vi "HP Values View.vi"(11 "Model in":refnum<class "Model.lvclass">) -> ()   [LabVIEW 2016, in "M1M3SupportEUI_Views.lvlib"]
uses:
  M1M3SupportEUI_Views.lvlib
  Model/Model.lvclass
  SALLV_m1m3/DataTypes/HardpointMonitorData.ctl
  SALLV_m1m3/DataTypes/HardpointActuatorData.ctl
  SALLV_m1m3/DataTypes/logevent_HardpointActuatorInfo.ctl
  SALLV_m1m3/DataTypes/logevent_HardpointMonitorInfo.ctl
  M1M3 Support Events/M1M3 Support Events.lvclass/M1M3 Support Events.ctl
  SALLV_m1m3/DataTypes/command_EnableHardpointCorrections.ctl
  SALLV_m1m3/DataTypes/command_DisableHardpointCorrections.ctl
  SALLV_m1m3/DataTypes/command_MoveHardpointActuators.ctl
  SALLV_m1m3/DataTypes/command_StopHardpointMotion.ctl
  SALLV_m1m3/DataTypes/command_EnableHardpointChase.ctl
  SALLV_m1m3/DataTypes/command_DisableHardpointChase.ctl
  SALLV_m1m3/DataTypes/command_PositionM1M3.ctl
  SALLV_m1m3/DataTypes/command_TranslateM1M3.ctl
  M1M3 Support Events/M1M3 Support Events.lvclass
  SALLV_m1m3/SALLV_m1m3.lvlib
  <vilib>/Utility/Data Type/NI_Data Type.lvlib
panel:
  out "T6":string
  out "T5":string
  out "T4":string
  out "T3":string
  out "T2":string
  out "T1":string
  out "ForceMagnitude":dbl
  out "E6":string
  out "E5":string
  out "E4":string
  out "E3":string
  out "E2":string
  out "E1":string
  out "Monitor Info Event Time Stamp":timestamp
  in  "MonitorInfoEvent":T1={"Timestamp"=0.0, "ReferenceId[6]"=[0, 0, 0, 0, 0, 0], "ModbusSubnet[6]"=[0, 0, 0, 0, 0, 0], "ModbusAddress[6]"=[0, 0, 0, 0, 0, 0], "ILCUniqueId[6]"=[0, 0, 0, 0, 0, 0], "ILCApplicationType[6]"=[0, 0, 0, 0, 0, 0], "NetworkNodeType[6]"=[0, 0, 0, 0, 0, 0], "MajorRevision[6]"=[0, 0, 0, 0, 0, 0], "MinorRevision[6]"=[0, 0, 0, 0, 0, 0], "MezzanineUniqueId[6]"=[0, 0, 0, 0, 0, 0], "MezzanineFirmwareType[6]"=[0, 0, 0, 0, 0, 0], "MezzanineMajorRevision[6]"=[0, 0, 0, 0, 0, 0], "MezzanineMinorRevision[6]"=[0, 0, 0, 0, 0, 0], "priority"=0}
  in  "Events Data Type":string(combo)
  in  "ActuatorInfoEvent":T2
  out "Z Magnitude":sgl
  out "Y Magnitude":sgl
  out "X Magnitude":sgl
  out "Z Force":sgl
  out "Y Force":sgl
  out "X Force":sgl
  in  "StopHardpointMotion":bool
  in  "HardpointMotionButton":bool
  in  "Input 6":i32
  in  "Input 5":i32
  in  "Input 4":i32
  in  "Input 3":i32
  in  "Input 2":i32
  in  "Input 1":i32
  in  "DisableHardpointCorrectionButton":bool
  in  "DisableHardpointChaseButton":bool
  in  "TranslateHardpointsButton":bool
  in  "PositionHardpointsButton":bool
  in  "Z Rotation Input":dbl
  in  "Y Rotation Input":dbl
  in  "X Rotation Input":dbl
  in  "Z Position Input":dbl
  in  "Y Position Input":dbl
  in  "X Position Input":dbl
  in  "EnableHardpointChaseButton":bool
  in  "EnableActuatorId":string(combo)
  in  "EnableHardpointCorrectionButton":bool
  out "Actuator Info Event Time Stamp":timestamp
  out "Z Rotation":sgl
  out "Y Rotation":sgl
  out "X Rotation":sgl
  out "Z Position":sgl
  out "Y Position":sgl
  out "X Position":sgl
  in  "HardpointActuatorData":T3={"Timestamp"=0.0, "StepsQueued[6]"=[0, 0, 0, 0, 0, 0], "StepsCommanded[6]"=[0, 0, 0, 0, 0, 0], "MeasuredForce[6]"=[0.0, 0.0, 0.0, 0.0, 0.0, 0.0], "Encoder[6]"=[0, 0, 0, 0, 0, 0], "Displacement[6]"=[0.0, 0.0, 0.0, 0.0, 0.0, 0.0], "Fx"=0.0, "Fy"=0.0, "Fz"=0.0, "Mx"=0.0, "My"=0.0, "Mz"=0.0, "ForceMagnitude"=0.0, "XPosition"=0.0, "YPosition"=0.0, "ZPosition"=0.0, "XRotation"=0.0, "YRotation"=0.0, "ZRotation"=0.0}
  in  "HardpointMonitorData":T4={"Timestamp"=0.0, "BreakawayLVDT[6]"=[0.0, 0.0, 0.0, 0.0, 0.0, 0.0], "DisplacementLVDT[6]"=[0.0, 0.0, 0.0, 0.0, 0.0, 0.0], "BreakawayPressure[6]"=[0.0, 0.0, 0.0, 0.0, 0.0, 0.0], "PressureSensor1[6]"=[0.0, 0.0, 0.0, 0.0, 0.0, 0.0], "PressureSensor2[6]"=[0.0, 0.0, 0.0, 0.0, 0.0, 0.0], "PressureSensor3[6]"=[0.0, 0.0, 0.0, 0.0, 0.0, 0.0]}
  out "Actuator Data Time Stamp":timestamp
  out "Monitor Data Time Stamp":timestamp
  in  "Telemetry Data Type":string(combo)
  # "Hardpoints"
  # "Events"
  # "Commands"
  # "Position"
  # "Rotation"
  # "X"
  # "3"
  # "1"
  # "2"
  # "Y"
  # "Z"
  # "6"
  # "4"
  # "5"
  # "Current Telemetry Values"
  # "Position (m)"
  # "Rotation (rad)"
  # "Force (N)"
  # "Moments(Nm)"
  # "3"
  # "1"
  # "2"
  # "X"
  # "6"
  # "4"
  # "5"
  # "Y"
  # "Z"
  # "3"
  # "1"
  # "2"
  # "6"
  # "4"
  # "5"
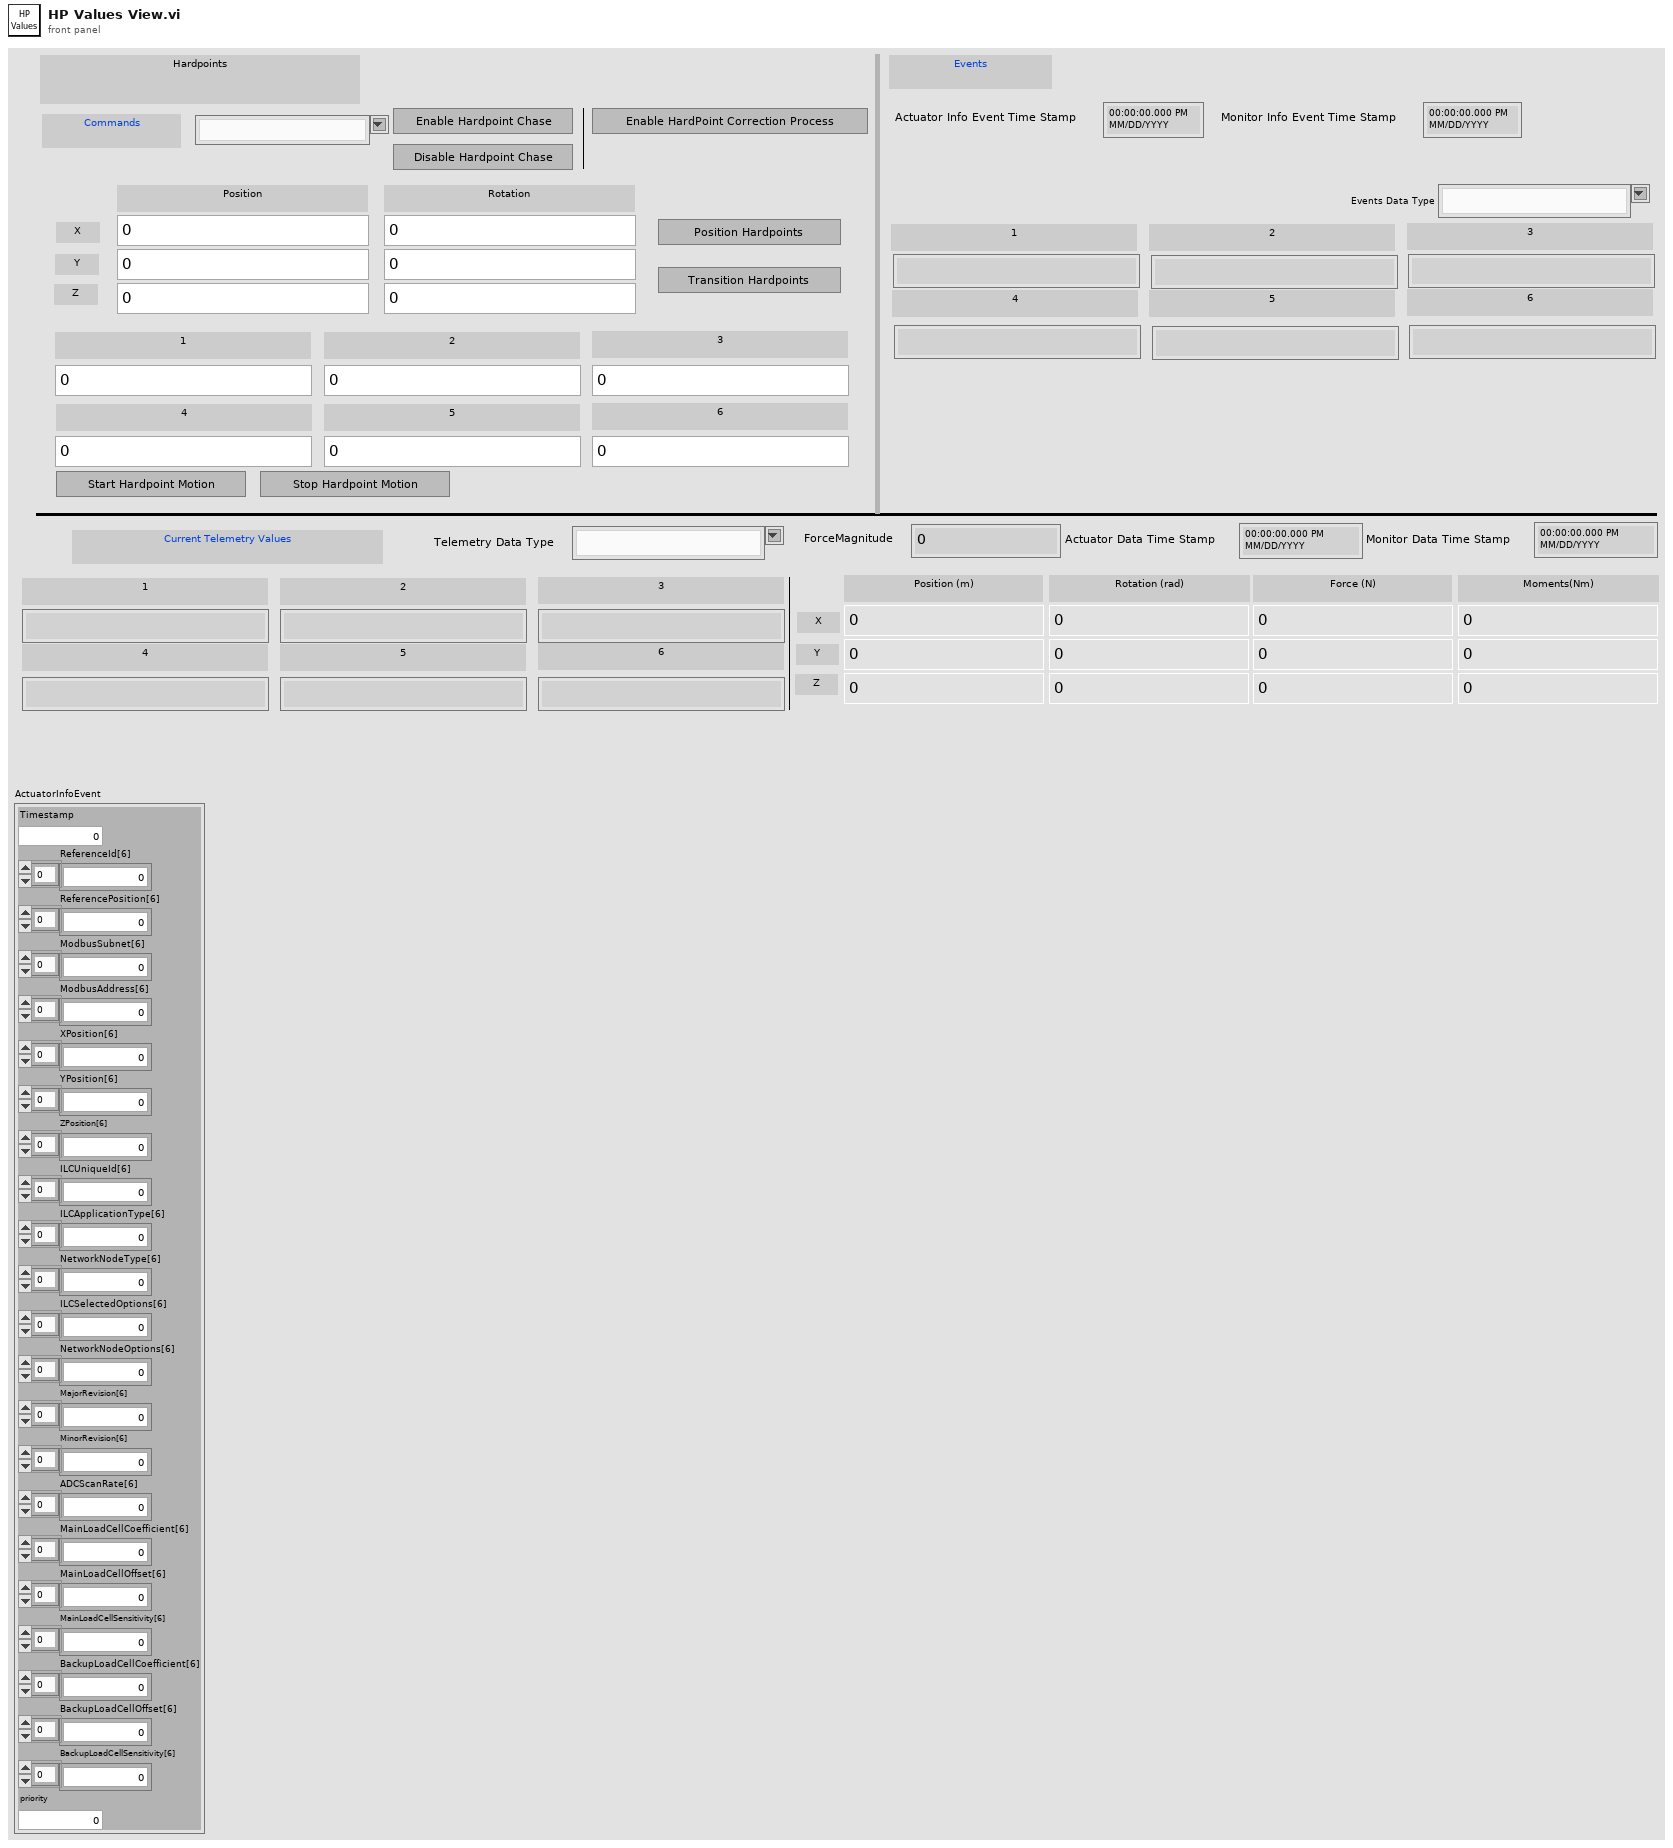
[diagram p1: front panel]
types:
  T1 = typedef "SALLV_m1m3.lvlib/logevent_HardpointMonitorInfo.ctl" = cluster{"Timestamp":dbl, "ReferenceId[6]":i16[], "ModbusSubnet[6]":i16[], "ModbusAddress[6]":i16[], "ILCUniqueId[6]":i64[], "ILCApplicationType[6]":i16[], "NetworkNodeType[6]":i16[], "MajorRevision[6]":i16[], "MinorRevision[6]":i16[], "MezzanineUniqueId[6]":i64[], "MezzanineFirmwareType[6]":i16[], "MezzanineMajorRevision[6]":i16[], "MezzanineMinorRevision[6]":i16[], "priority":i32}
  T2 = typedef "SALLV_m1m3.lvlib/logevent_HardpointActuatorInfo.ctl" = cluster{"Timestamp":dbl, "ReferenceId[6]":i16[], "ReferencePosition[6]":i32[], "ModbusSubnet[6]":i16[], "ModbusAddress[6]":i16[], "XPosition[6]":sgl[], "YPosition[6]":sgl[], "ZPosition[6]":sgl[], "ILCUniqueId[6]":i64[], "ILCApplicationType[6]":i16[], "NetworkNodeType[6]":i16[], "ILCSelectedOptions[6]":i16[], "NetworkNodeOptions[6]":i16[], "MajorRevision[6]":i16[], "MinorRevision[6]":i16[], "ADCScanRate[6]":i16[], "MainLoadCellCoefficient[6]":sgl[], "MainLoadCellOffset[6]":sgl[], "MainLoadCellSensitivity[6]":sgl[], "BackupLoadCellCoefficient[6]":sgl[], "BackupLoadCellOffset[6]":sgl[], "BackupLoadCellSensitivity[6]":sgl[], "priority":i32}
  T3 = typedef "SALLV_m1m3.lvlib/HardpointActuatorData.ctl" = cluster{"Timestamp":dbl, "StepsQueued[6]":i32[], "StepsCommanded[6]":i16[], "MeasuredForce[6]":sgl[], "Encoder[6]":i32[], "Displacement[6]":sgl[], "Fx":sgl, "Fy":sgl, "Fz":sgl, "Mx":sgl, "My":sgl, "Mz":sgl, "ForceMagnitude":sgl, "XPosition":sgl, "YPosition":sgl, "ZPosition":sgl, "XRotation":sgl, "YRotation":sgl, "ZRotation":sgl}
  T4 = typedef "SALLV_m1m3.lvlib/HardpointMonitorData.ctl" = cluster{"Timestamp":dbl, "BreakawayLVDT[6]":sgl[], "DisplacementLVDT[6]":sgl[], "BreakawayPressure[6]":sgl[], "PressureSensor1[6]":sgl[], "PressureSensor2[6]":sgl[], "PressureSensor3[6]":sgl[]}
  T5 = enum16{"", "DetailedState_DetailedStates_DisabledState", "DetailedState_DetailedStates_EnabledState", "DetailedState_DetailedStates_FaultState", "DetailedState_DetailedStates_OfflineState", "DetailedState_DetailedStates_StandbyState", "DetailedState_DetailedStates_ParkedState", "DetailedState_DetailedStates_RaisingState", "DetailedState_DetailedStates_ActiveState", "DetailedState_DetailedStates_LoweringState", "DetailedState_DetailedStates_EngineeringState", "DetailedState_DetailedStates_ParkedEngineeringState", "DetailedState_DetailedStates_RaisingEngineeringState", "DetailedState_DetailedStates_ActiveEngineeringState", "DetailedState_DetailedStates_LoweringEngineeringState", "DetailedState_DetailedStates_LoweringFaultState", "DetailedState_DetailedStates_ProfileHardpointCorrectionState"}
  T6 = typedef "M1M3SupportEUI_TypeDefs.lvlib/M1M3 Support Events.ctl" = cluster{"Inclinometer  Data":refnum<user-event>, "IMS Data":refnum<user-event>, "SAL Connected":refnum<user-event>, "Accelerometer Data":refnum<user-event>, "OuterLoop Data":refnum<user-event>, "ErrorCode Event":refnum<user-event>, "InterlockStatus Event":refnum<user-event>, "InterlockWarning Event":refnum<user-event>, "Gyro Data":refnum<user-event>, "HP Actuator Info Event":refnum<user-event>, " FA Info Event":refnum<user-event>, "HP Monitor Info Event":refnum<user-event>, "FA Data":refnum<user-event>, "HP Actuator data":refnum<user-event>, "HP Monitor data":refnum<user-event>, "Air Supply Status Event":refnum<user-event>, "Air Supply Warning Event":refnum<user-event>, "Power Data":refnum<user-event>, "PID Data":refnum<user-event>, "PID Info Event":refnum<user-event>, "Power Status Event":refnum<user-event>, "Power Supply Status Event":refnum<user-event>, "Power Warning Event":refnum<user-event>, "Summary State Event":refnum<user-event>, "Detailed State Event":refnum<user-event>, "FA Force Warning Event":refnum<user-event>, "FA Warning Event":refnum<user-event>, "FA State Event":refnum<user-event>, "Applied AberrationForces Event":refnum<user-event>, "Applied Acceleration Forcces Event":refnum<user-event>, "Applied Azimuth Forces Event":refnum<user-event>, "Applied Active Optic Forces Event":refnum<user-event>, "Applied Balance Forces Event":refnum<user-event>, "Applied Cylinder Forces Event":refnum<user-event>, "Applied Elevation Forces Event":refnum<user-event>, "Applied Forces Event":refnum<user-event>, "Applied Offset Forces Event":refnum<user-event>, "Applied Static Forces Event":refnum<user-event>, "Applied Thermal Forces Event":refnum<user-event>, "Applied Velocity Forces Event":refnum<user-event>, "Rejected Aberration Force Event":refnum<user-event>, "Rejected Acceleration Forces Event":refnum<user-event>, "Rejected Active Optic Forces Event":refnum<user-event>, "Rejected Azimuth Forces Event":refnum<user-event>, "Rejected Balance Forces Event":refnum<user-event>, "Rejected Cylinder Forces Event":refnum<user-event>, "Rejected Elevation Forces Event":refnum<user-event>, "Rejected Forces Event":refnum<user-event>, "Rejected Offset Forces Event":refnum<user-event>, "Rejected Static Forces Event":refnum<user-event>, "Rejected Thermal Forces Event":refnum<user-event>, "Rejected Velocity Forces Event":refnum<user-event>, "Command Rejection Event":refnum<user-event>, "Setting Verions Event":refnum<user-event>, "Settings Applied Event":refnum<user-event>}
  T7 = typedef "NI_Data Type.lvlib/Data Type.ctl" = enum8{"Invalid Type", "Void", "I8", "I16", "I32", "I64", "U8", "U16", "U32", "U64", "Single Float", "Double Float", "Extended Float", "Single Complex", "Double Complex", "Extended Complex", "Enum U8", "Enum U16", "Enum U32", "Enum U64", "Single Float With Unit", "Double Float With Unit", "Extended Float With Unit", "Single Complex with Unit", "Double Complex with Unit", "Extended Complex with Unit", "Boolean", "String", "Path", "Picture", "Tag", "Array", "Cluster", "Variant", "LV Variant", "Waveform", "Timestamp", "Digital Waveform", "Digital Data", "ExpressData", "Refnum", "External Data", "VI", "Poly VI", "LabVIEW Class Instance", "Fixed Point"}
  T8 = typedef "SALLV_m1m3.lvlib/command_EnableHardpointCorrections.ctl" = cluster{"EnableHardpointCorrections":bool}
  T9 = typedef "SALLV_m1m3.lvlib/command_DisableHardpointCorrections.ctl" = cluster{"DisableHardpointCorrections":bool}
  T10 = typedef "SALLV_m1m3.lvlib/command_MoveHardpointActuators.ctl" = cluster{"Steps[6]":i32[]}
  T11 = typedef "SALLV_m1m3.lvlib/command_StopHardpointMotion.ctl" = cluster{"StopHardpointMotion":bool}
  T12 = typedef "SALLV_m1m3.lvlib/command_EnableHardpointChase.ctl" = cluster{"HardpointActuator":i16}
  T13 = typedef "SALLV_m1m3.lvlib/command_DisableHardpointChase.ctl" = cluster{"HardpointActuator":i16}
  T14 = typedef "SALLV_m1m3.lvlib/command_PositionM1M3.ctl" = cluster{"XPosition":sgl, "YPosition":sgl, "ZPosition":sgl, "XRotation":sgl, "YRotation":sgl, "ZRotation":sgl}
  T15 = typedef "SALLV_m1m3.lvlib/command_TranslateM1M3.ctl" = cluster{"XTranslation":sgl, "YTranslation":sgl, "ZTranslation":sgl, "XRotation":sgl, "YRotation":sgl, "ZRotation":sgl}
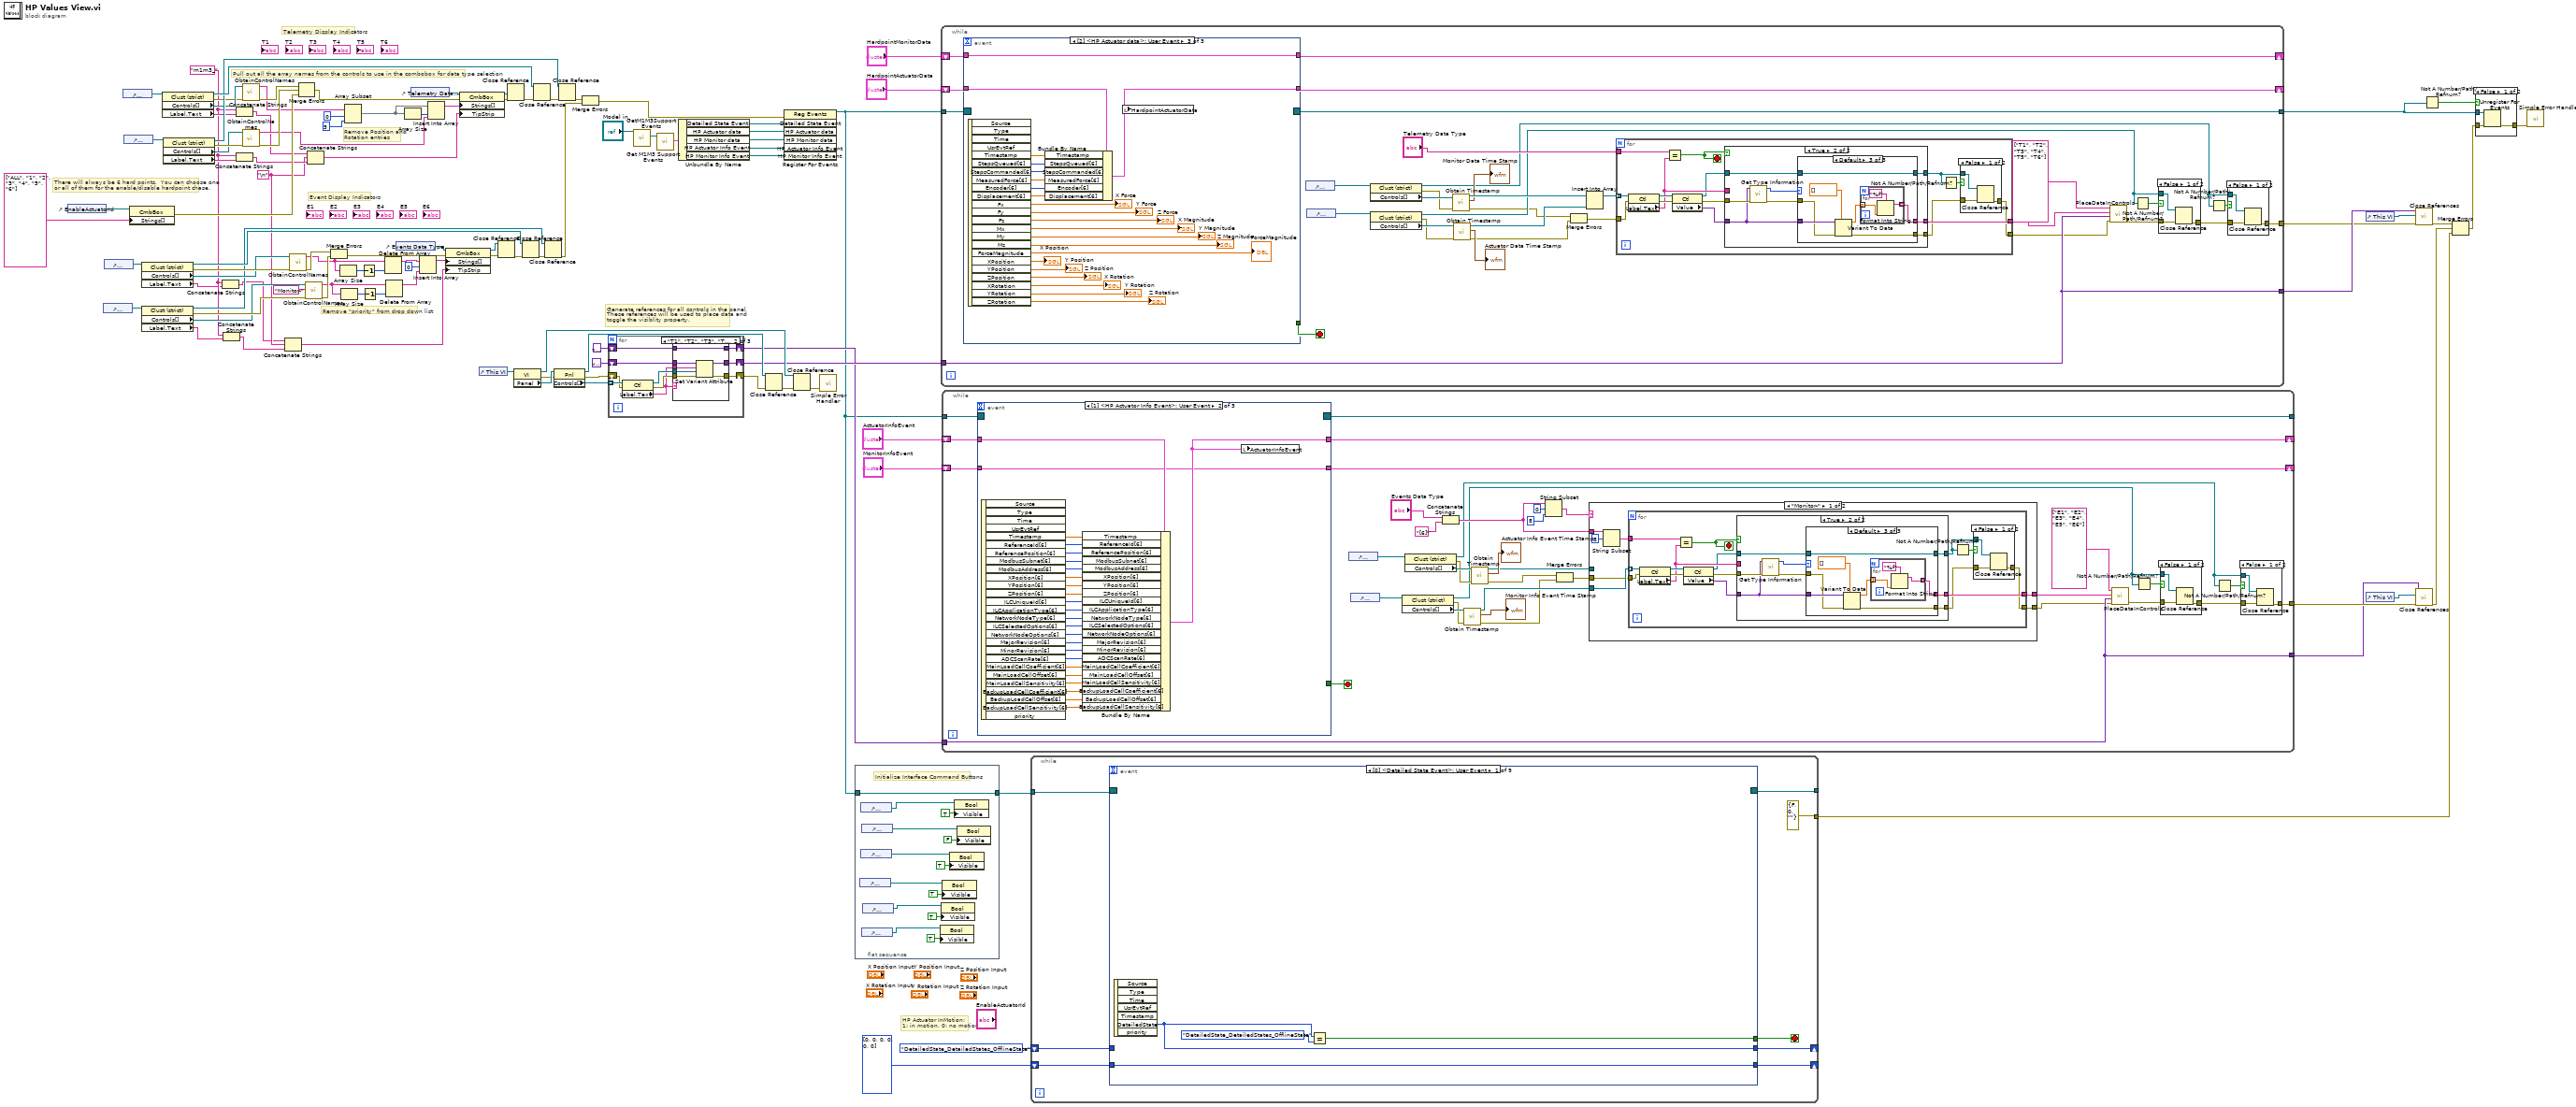
[diagram p0: block diagram]
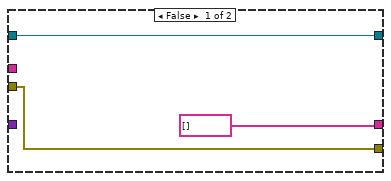
[diagram p4: hidden frame]
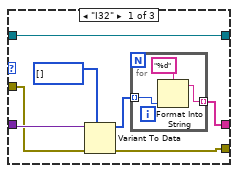
[diagram p5: hidden frame]
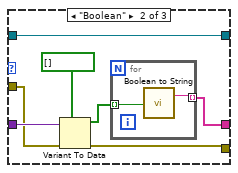
[diagram p6: hidden frame]
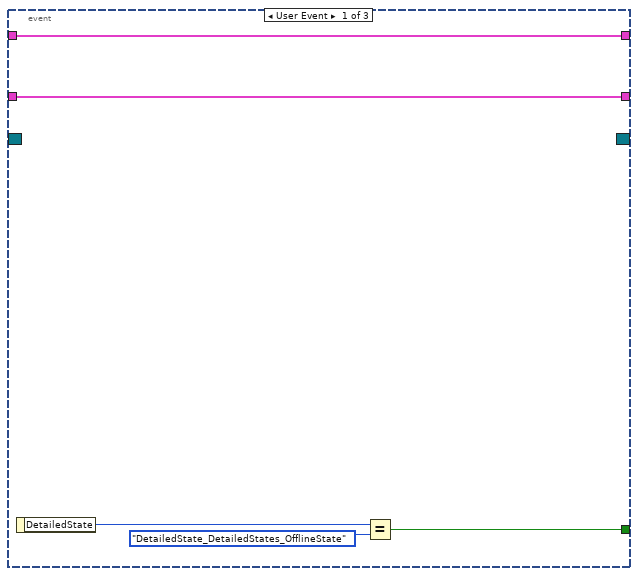
[diagram p7: hidden frame]
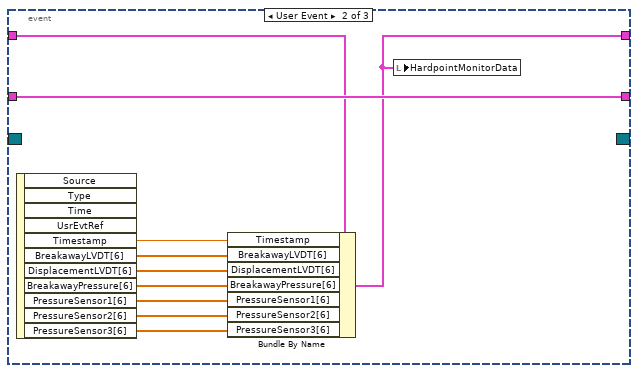
[diagram p8: hidden frame]
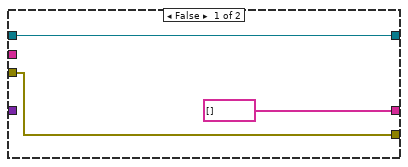
[diagram p11: hidden frame]
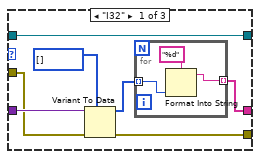
[diagram p12: hidden frame]
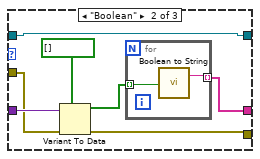
[diagram p13: hidden frame]
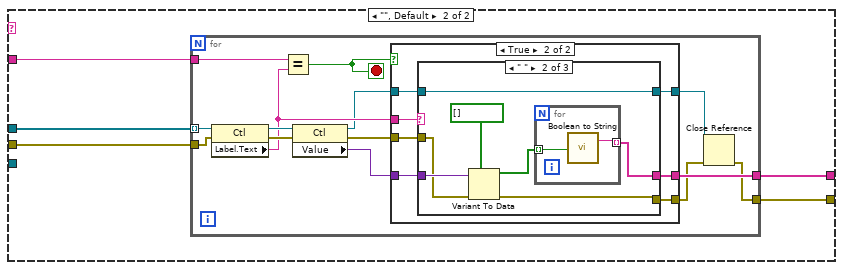
[diagram p15: hidden frame]
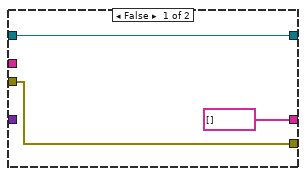
[diagram p16: hidden frame]
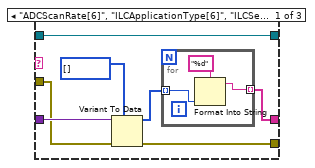
[diagram p17: hidden frame]
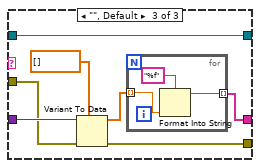
[diagram p18: hidden frame]
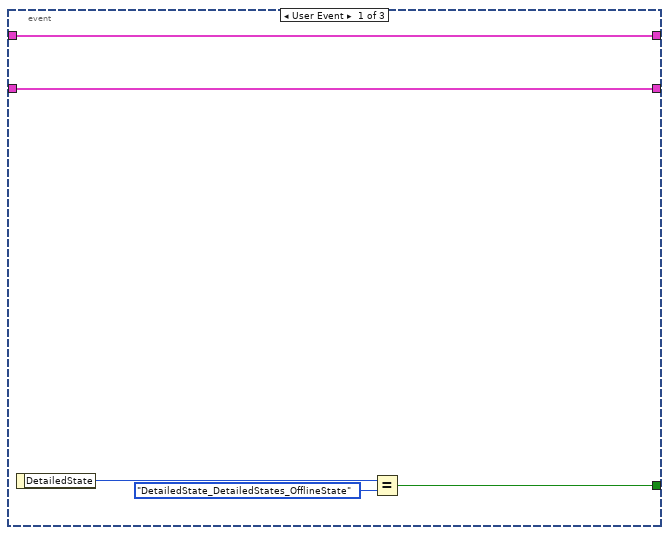
[diagram p19: hidden frame]
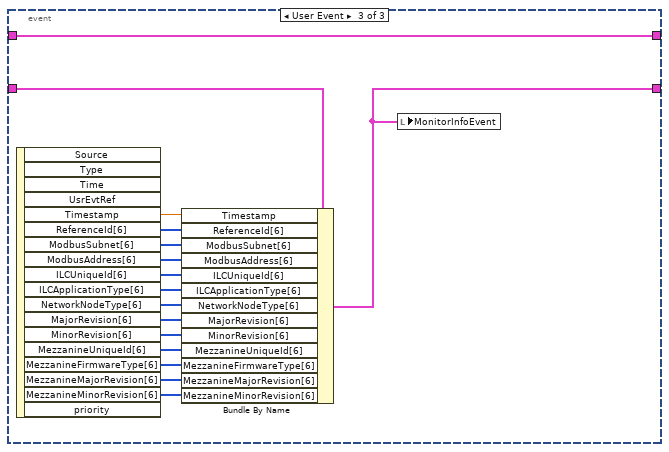
[diagram p20: hidden frame]
diagram:
  w4 = "\n"
  w8 = "m1m3_"
  # "Remove \"priority\" from drop down list"
  # "Event Display Indicators"
  # "Telemetry Display Indicators"
  # "HP Actuator InMotion:\n1: in motion, 0: no motion"
  # "There will always be 6 hard points.  You can choose one\nor all of them for the enable/disable hardpoint chase."
  # "Remove Position and\nRotation entries"
  # "Generate references for all controls in the panel\nThese references will be used to place data and\ntoggle the visiblity property."
  # "Pull out all the array names from the controls to use in the combobox for data type selection"
  n1 = control-ref of="EnableActuatorId"() -> (w83:refnum<vi>)
  n2 = control-ref of="MonitorInfoEvent"() -> (w50:refnum<vi>)
  n3 = control-ref of="ActuatorInfoEvent"() -> (w76:refnum<vi>)
  n4 = control-ref of="HardpointActuatorData"() -> (w66:refnum<vi>)
  n5 = control-ref of="HardpointMonitorData"() -> (w65:refnum<vi>)
  n6 = property class="CmbBox"(reference=w83, "Strings[]"=string[] ["ALL", "1", "2", "3", "4", "5", "6"]) -> (error out=w81:errorcluster)  [unwired: 1 in, 1 out]
  n7 = property class="Clust (strict)"(reference=w76) -> (reference out=w72:refnum<vi>, error out=w56:errorcluster, "Controls[]"=w55:refnum<vi>[], "Label.Text"=w7:string)  [unwired: 1 in]
  n8 = property class="Clust (strict)"(reference=w50) -> (reference out=w47:refnum<vi>, error out=w51:errorcluster, "Controls[]"=w49:refnum<vi>[], "Label.Text"=w6:string)  [unwired: 1 in]
  n9 = property class="Clust (strict)"(reference=w66) -> (reference out=w106:refnum<vi>, error out=w63:errorcluster, "Controls[]"=w64:refnum<vi>[], "Label.Text"=w12:string)  [unwired: 1 in]
  n10 = property class="Clust (strict)"(reference=w65) -> (reference out=w101:refnum<vi>, error out=w61:errorcluster, "Controls[]"=w60:refnum<vi>[], "Label.Text"=w11:string)  [unwired: 1 in]
  n11 = Concatenate Strings(w8, w7) -> (w3:string)
  n12 = Concatenate Strings(w8, w6) -> (w2:string)
  n13 = Concatenate Strings(w8, w12) -> (w10:string)
  n14 = Concatenate Strings(w8, w11) -> (w5:string)
  n15 = call "ObtainControlNames.vi"("error in (no error)"=w63, "ControlRefnumArray"=w64) -> ("error out"=w62:errorcluster, "ControlNamesArray"=w33:string[])  [unwired: 8 in]
  n16 = call "ObtainControlNames.vi"("error in (no error)"=w61, "ControlRefnumArray"=w60) -> ("error out"=w59:errorcluster, "ControlNamesArray"=w58:string[])  [unwired: 8 in]
  n17 = Concatenate Strings(w3, w4, w2) -> (w1:string)
  n18 = call "ObtainControlNames.vi"("error in (no error)"=w56, "ControlRefnumArray"=w55) -> ("error out"=w54:errorcluster, "ControlNamesArray"=w41:string[])  [unwired: 8 in]
  n19 = Merge Errors(w62, w59, w81) -> (w105:errorcluster)
  n20 = call "ObtainControlNames.vi"("error in (no error)"=w51, "AddedPrefix"="Monitor-", "ControlRefnumArray"=w49) -> ("error out"=w46:errorcluster, "ControlNamesArray"=w35:string[])  [unwired: 7 in]
  n21 = Concatenate Strings(w10, w4, w5) -> (w9:string)
  n22 = Merge Errors(w54, w46) -> (w73:errorcluster)
  n23 = Array Size(array=w41) -> (size(s)=w40:i32)
  n24 = Array Size(array=w35) -> (size(s)=w36:i32)
  n25 = Array Subset(array=w33, index=0, length=5 ("y")) -> (w32:string[])
  n26 = Decrement(x=w40) -> (x-1=w39:i32)
  n27 = Decrement(x=w36) -> (x-1=w37:i32)
  n28 = Delete From Array(array=w41, index=w39) -> (array with subset deleted=w38:string[])  [unwired: 1 in, 1 out]
  n29 = Delete From Array(array=w35, index=w37) -> (array with subset deleted=w34:string[])  [unwired: 1 in, 1 out]
  n30 = control-ref of="Events Data Type"() -> (w74:refnum<vi>)
  n31 = Array Size(array=w32) -> (size(s)=w85:i32)
  n32 = control-ref of="Telemetry Data Type"() -> (w100:refnum<vi>)
  n33 = Insert Into Array(array=w38, index=0, new element=w34) -> (w52:string[])
  n34 = Insert Into Array(array=w32, index=w85, new element=w58) -> (w102:string[])
  n35 = property class="CmbBox"(reference=w74, error in=w73, "Strings[]"=w52, "TipStrip"=w1) -> (reference out=w27:refnum<vi>, error out=w26:errorcluster)
  n36 = property class="CmbBox"(reference=w100, error in=w105, "Strings[]"=w102, "TipStrip"=w9) -> (reference out=w29:refnum<vi>, error out=w28:errorcluster)
  n37 = control-ref of="This VI"() -> (w87:refnum<vi>)
  n38 = Close Reference(reference=w27, error in (no error)=w26) -> (error out=w57:errorcluster)
  n39 = Close Reference(reference=w29, error in (no error)=w28) -> (error out=w103:errorcluster)
  n40 = property class="VI"(reference=w87) -> (reference out=w97:refnum<vi>, error out=w88:errorcluster, "Panel"=w89:refnum<vi>)  [unwired: 1 in]
  n41 = Close Reference(reference=w72, error in (no error)=w57) -> (error out=w48:errorcluster)
  n42 = Close Reference(reference=w106, error in (no error)=w103) -> (error out=w104:errorcluster)
  n43 = Close Reference(reference=w47, error in (no error)=w48) -> (error out=w43:errorcluster)
  n44 = property class="Pnl"(reference=w89, error in=w88) -> (reference out=w95:refnum<vi>, error out=w92:errorcluster, "Controls[]"=w90:refnum<vi>[])
  n45 = Close Reference(reference=w101, error in (no error)=w104) -> (error out=w45:errorcluster)
  n46 = Merge Errors(w45, w43) -> (w44:errorcluster)
  n47 = for {
    tunnel: w90 -> [w121] mode=indexing
    shift-right: [w118] -> w77
    shift-left: variant -> [w120]
    shift-right: [w115] -> w94
    shift-left: w92 -> [w117]
    shift-right: [w113] -> w71
    shift-left: variant -> [w114]
    n48 = property class="Ctl"(reference=w121, error in=w117) -> (reference out=w119:refnum<vi>, error out=w116:errorcluster, "Label.Text"=w112:string)
    n49 = case shown="\"T1\", \"T2\", \"T3\", \"T4\", \"T5\", \"T6\"" w112 {
      tunnel: w120 -> [w123 w131 w136]
      tunnel: w112 -> [_ w130 w135]
      tunnel: w119 -> [_ w129 w134]
      tunnel: [w123 w128 w136] -> w118
      tunnel: w116 -> [w122 w127 w133]
      tunnel: [w122 w126 w132] -> w115
      tunnel: w114 -> [w124 w125 w138]
      tunnel: [w124 w125 w137] -> w113
      frame "", Default {
      }
      frame "T1", "T2", "T3", "T4", "T5", "T6" {
        n50 = Set Variant Attribute(Variant=w131, name=w130, value=w129, error in=w127) -> (Variant out=w128:variant, error out=w126:errorcluster)  [unwired: 1 out]
      }
      frame "E1", "E2", "E3", "E4", "E5", "E6" {
        n51 = Set Variant Attribute(Variant=w138, name=w135, value=w134, error in=w133) -> (Variant out=w137:variant, error out=w132:errorcluster)  [unwired: 1 out]
      }
    }
  }
  n52 = call "GetM1M3SupportEvents.vi"("Model in"="Model in") -> ("M1M3 Support Events out"=w111:refnum<class "M1M3 Support Events.lvclass">)  [unwired: 8 in, 2 out]
  n53 = call "Get M1M3 Support Events.vi"("M1M3 Support Events in"=w111) -> ("M1M3 Support Events"=w110:T6)  [unwired: 9 in, 1 out]
  n54 = Unbundle By Name(w110) -> ("Detailed State Event"=w108:refnum<user-event>, "HP Actuator data"=w107:refnum<user-event>, "HP Monitor data"=w86:refnum<user-event>, "HP Actuator Info Event"=w84:refnum<user-event>, "HP Monitor Info Event"=w80:refnum<user-event>)
  n55 = Close Reference(reference=w95, error in (no error)=w94) -> (error out=w93:errorcluster)
  n56 = register-events(error in=w44, w108, w107, w86, w84, w80) -> (reference out=w70:refnum<event-registration>)  [unwired: 1 in, 1 out]
  n57 = Close Reference(reference=w97, error in (no error)=w93) -> (error out=w96:errorcluster)
  n58 = call <vilib>:"Simple Error Handler.vi"("error in (no error)"=w96) -> ()  [unwired: 4 in, 5 out]
  n59 = flat-sequence {
    tunnel: [w151] -> w78
    tunnel: w70 -> [w151]
    frame #0 {
      # "Initialize Interface Command Buttons"
      n60 = control-ref of="DisableHardpointChaseButton"() -> (w139:refnum<vi>)
      n61 = control-ref of="EnableHardpointCorrectionButton"() -> (w144:refnum<vi>)
      n62 = control-ref of="EnableHardpointChaseButton"() -> (w141:refnum<vi>)
      n63 = control-ref of="StopHardpointMotion"() -> (w148:refnum<vi>)
      n64 = control-ref of="DisableHardpointCorrectionButton"() -> (w143:refnum<vi>)
      n65 = control-ref of="HardpointMotionButton"() -> (w147:refnum<vi>)
      n66 = property class="Bool"(reference=w148, "Visible"=TRUE) -> ()  [unwired: 1 in, 2 out]
      n67 = property class="Bool"(reference=w147, "Visible"=TRUE) -> ()  [unwired: 1 in, 2 out]
      n68 = property class="Bool"(reference=w139, "Visible"=TRUE) -> ()  [unwired: 1 in, 2 out]
      n69 = property class="Bool"(reference=w141, "Visible"=TRUE) -> ()  [unwired: 1 in, 2 out]
      n70 = property class="Bool"(reference=w144, "Visible"=TRUE) -> ()  [unwired: 1 in, 2 out]
      n71 = property class="Bool"(reference=w143, "Visible"=FALSE) -> ()  [unwired: 1 in, 2 out]
    }
  }
  n72 = while {
    tunnel: w70 -> [w184]
    shift-right: [w181] -> _
    shift-left: "HardpointMonitorData" -> [w182]
    shift-right: [w179] -> _
    shift-left: "HardpointActuatorData" -> [w180]
    tunnel: w77 -> [w162]
    tunnel: [w162] -> w25
    tunnel: [w176] -> w17
    tunnel: [w156] -> w19
    stop <- w183 stop-if-true
    n73 = event shown="[2] <HP Actuator data>: User Event" {
      selector: w184 -> [_ _ _]
      dyn-events: [_ _ _] -> w176
      timeout: _ -> [_ _ _]
      tunnel: [w248 _ _] -> w183
      tunnel: w182 -> [w247 w257 w280]
      tunnel: [w247 w256 w280] -> w181
      tunnel: w180 -> [w246 w258 w279]
      tunnel: [w246 w258 w278] -> w179
      event User Event {
        n74 = event-data() -> ("DetailedState"=w245:T5)  [unwired: 1 in]
        n75 = Equal?(x=w245, y=T5."DetailedState_DetailedStates_OfflineState") -> (x = y?=w248:bool)
      }
      event User Event {
        n76 = event-data() -> ("Timestamp"=w255:dbl, "BreakawayLVDT[6]"=w254:sgl[], "DisplacementLVDT[6]"=w253:sgl[], "BreakawayPressure[6]"=w252:sgl[], "PressureSensor1[6]"=w251:sgl[], "PressureSensor2[6]"=w250:sgl[], "PressureSensor3[6]"=w249:sgl[])  [unwired: 1 in, 4 out]
        n77 = Bundle By Name(cluster=w257, "Timestamp"=w255, "BreakawayLVDT[6]"=w254, "DisplacementLVDT[6]"=w253, "BreakawayPressure[6]"=w252, "PressureSensor1[6]"=w251, "PressureSensor2[6]"=w250, "PressureSensor3[6]"=w249) -> (w256:T4)
        n78 = local write "HardpointMonitorData"(w256) -> ()
      }
      event User Event {
        n79 = event-data() -> ("Timestamp"=w277:dbl, "StepsQueued[6]"=w276:i32[], "StepsCommanded[6]"=w275:i16[], "MeasuredForce[6]"=w274:sgl[], "Encoder[6]"=w273:i32[], "Displacement[6]"=w272:sgl[], "Fx"=→"X Force":sgl, "Fy"=→"Y Force":sgl, "Fz"=→"Z Force":sgl, "Mx"=→"X Magnitude":sgl, "My"=→"Y Magnitude":sgl, "Mz"=→"Z Magnitude":sgl, "ForceMagnitude"=→"ForceMagnitude":sgl, "XPosition"=→"X Position":sgl, "YPosition"=→"Y Position":sgl, "ZPosition"=→"Z Position":sgl, "XRotation"=→"X Rotation":sgl, "YRotation"=→"Y Rotation":sgl, "ZRotation"=→"Z Rotation":sgl)  [unwired: 1 in, 4 out]
        n80 = Bundle By Name(cluster=w279, "Timestamp"=w277, "StepsQueued[6]"=w276, "StepsCommanded[6]"=w275, "MeasuredForce[6]"=w274, "Encoder[6]"=w273, "Displacement[6]"=w272) -> (w278:T3)
        n81 = local write "HardpointActuatorData"(w278) -> ()
      }
    }
    n82 = control-ref of="HardpointMonitorData"() -> (w178:refnum<vi>)
    n83 = control-ref of="HardpointActuatorData"() -> (w177:refnum<vi>)
    n84 = property class="Clust (strict)"(reference=w178) -> (reference out=w157:refnum<vi>, error out=w171:errorcluster, "Controls[]"=w173:refnum<vi>[])  [unwired: 1 in]
    n85 = property class="Clust (strict)"(reference=w177) -> (reference out=w160:refnum<vi>, error out=w169:errorcluster, "Controls[]"=w170:refnum<vi>[])  [unwired: 1 in]
    n86 = call "Obtain Timestamp.vi"("error in (no error)"=w171, "ControlRefnumArray"=w173) -> ("error out"=w154:errorcluster, "Time Stamp"=→"Monitor Data Time Stamp":timestamp, "Array"=w172:refnum<vi>[])  [unwired: 7 in]
    n87 = call "Obtain Timestamp.vi"("error in (no error)"=w169, "ControlRefnumArray"=w170) -> ("error out"=w153:errorcluster, "Time Stamp"=→"Actuator Data Time Stamp":timestamp, "Array"=w166:refnum<vi>[])  [unwired: 7 in]
    n88 = Merge Errors(w154, w153) -> (w152:errorcluster)
    n89 = Insert Into Array(array=w172, new element=w166) -> (w174:refnum<vi>[])  [unwired: 1 in]
    n90 = for {
      tunnel: "Telemetry Data Type" -> [w193]
      tunnel: w174 -> [w198] mode=indexing
      tunnel: [w191] -> w164
      tunnel: [w186] -> w155
      tunnel: w152 -> [w185]
      stop <- w195 stop-if-true
      n91 = property class="Ctl"(reference=w198, error in=w185) -> (reference out=w196:refnum<vi>, error out=w197:errorcluster, "Label.Text"=w192:string)
      n92 = Equal?(x=w193, y=w192) -> (x = y?=w195:bool)
      n93 = property class="Ctl"(reference=w196, error in=w197) -> (reference out=w190:refnum<vi>, error out=w194:errorcluster, "Value"=w199:variant)
      n94 = case shown="True" w195 {
        tunnel: w199 -> [_ w208]
        tunnel: w192 -> [_ _]
        tunnel: w194 -> [w206 w210]
        tunnel: [w206 w214] -> w187
        tunnel: [string[] [] w213] -> w191
        tunnel: w190 -> [w204 w212]
        tunnel: [w204 w211] -> w188
        frame False {
        }
        frame True {
          n95 = call <vilib>:"Get Type Information.vi"("error in (no error)"=w210, "Variant"=w208) -> ("error out"=w209:errorcluster, "Type"=w207:T7)  [unwired: 5 in, 3 out]
          n96 = case shown="Default" w207 {
            tunnel: w208 -> [w220 w230 w240]
            tunnel: [w216 w226 w235] -> w213
            tunnel: w209 -> [w219 w229 w238]
            tunnel: [w218 w228 w237] -> w214
            tunnel: w212 -> [w215 w225 w234]
            tunnel: [w215 w225 w234] -> w211
            frame "I32" {
              n97 = Variant To Data(error in=w219, type=i32[] [], Variant=w220) -> (data=w217:i32[], error out=w218:errorcluster)
              n98 = for {
                tunnel: w217 -> [w224] mode=indexing
                tunnel: [w223] -> w216 mode=indexing
                n99 = Format Into String(format string="%d", w224) -> (resulting string=w223:string)  [unwired: 2 in, 1 out]
              }
            }
            frame "Boolean" {
              n100 = Variant To Data(error in=w229, type=bool[] [], Variant=w230) -> (data=w227:bool[], error out=w228:errorcluster)
              n101 = for {
                tunnel: w227 -> [w233] mode=indexing
                tunnel: [w232] -> w226 mode=indexing
                n102 = call "Boolean to String.vi"("BooleanValue"=w233) -> ("StringForm"=w232:string)  [unwired: 1 out]
              }
            }
            frame Default {
              n103 = Variant To Data(error in=w238, type=dbl[] [], Variant=w240) -> (data=w236:dbl[], error out=w237:errorcluster)
              n104 = for {
                tunnel: w236 -> [w243] mode=indexing
                tunnel: [w242] -> w235 mode=indexing
                n105 = Format Into String(format string="%f", w243) -> (resulting string=w242:string)  [unwired: 2 in, 1 out]
              }
            }
          }
        }
      }
      n106 = Not A Number/Path/Refnum?(number/path/refnum=w188) -> (NaN/Path/Refnum?=w189:bool)
      n107 = case shown="False" w189 {
        tunnel: w187 -> [w202 w203]
        tunnel: [w201 w203] -> w186
        tunnel: w188 -> [w200 _]
        frame False {
          n108 = Close Reference(reference=w200, error in (no error)=w202) -> (error out=w201:errorcluster)
        }
        frame True {
        }
      }
    }
    n109 = call "PlaceDataInControls.vi"("error in (no error)"=w155, "Variant"=w162, "DataArray"=w164, "ControlNamesArray"=string[] ["T1", "T2", "T3", "T4", "T5", "T6"]) -> ("error out"=w161:errorcluster)  [unwired: 7 in]
    n110 = Not A Number/Path/Refnum?(number/path/refnum=w160) -> (NaN/Path/Refnum?=w163:bool)
    n111 = case shown="False" w163 {
      tunnel: w161 -> [w283 w284]
      tunnel: [w282 w284] -> w158
      tunnel: w160 -> [w281 _]
      frame False {
        n112 = Close Reference(reference=w281, error in (no error)=w283) -> (error out=w282:errorcluster)
      }
      frame True {
      }
    }
    n113 = Not A Number/Path/Refnum?(number/path/refnum=w157) -> (NaN/Path/Refnum?=w159:bool)
    n114 = case shown="False" w159 {
      tunnel: w158 -> [w287 w288]
      tunnel: [w286 w288] -> w156
      tunnel: w157 -> [w285 _]
      frame False {
        n115 = Close Reference(reference=w285, error in (no error)=w287) -> (error out=w286:errorcluster)
      }
      frame True {
      }
    }
  }
  n116 = while {
    tunnel: w71 -> [w307]
    tunnel: w70 -> [w325]
    shift-right: [w322] -> _
    shift-left: "ActuatorInfoEvent" -> [w323]
    shift-right: [w317] -> _
    shift-left: "MonitorInfoEvent" -> [w318]
    tunnel: [w295] -> w22
    tunnel: [w307] -> w21
    tunnel: [w289] -> _
    stop <- w324 stop-if-true
    n117 = event shown="[1] <HP Actuator Info Event>: User Event" {
      selector: w325 -> [_ _ _]
      dyn-events: [_ _ _] -> w289
      timeout: _ -> [_ _ _]
      tunnel: [w454 _ _] -> w324
      tunnel: w323 -> [w453 w479 w495]
      tunnel: [w453 w478 w495] -> w322
      tunnel: w318 -> [w452 w455 w494]
      tunnel: [w452 w455 w493] -> w317
      event User Event {
        n118 = event-data() -> ("DetailedState"=w451:T5)  [unwired: 1 in]
        n119 = Equal?(x=w451, y=T5."DetailedState_DetailedStates_OfflineState") -> (x = y?=w454:bool)
      }
      event User Event {
        n120 = event-data() -> ("Timestamp"=w477:dbl, "ReferenceId[6]"=w476:i16[], "ReferencePosition[6]"=w475:i32[], "ModbusSubnet[6]"=w474:i16[], "ModbusAddress[6]"=w473:i16[], "XPosition[6]"=w472:sgl[], "YPosition[6]"=w471:sgl[], "ZPosition[6]"=w470:sgl[], "ILCUniqueId[6]"=w469:i64[], "ILCApplicationType[6]"=w468:i16[], "NetworkNodeType[6]"=w467:i16[], "ILCSelectedOptions[6]"=w466:i16[], "NetworkNodeOptions[6]"=w465:i16[], "MajorRevision[6]"=w464:i16[], "MinorRevision[6]"=w463:i16[], "ADCScanRate[6]"=w462:i16[], "MainLoadCellCoefficient[6]"=w461:sgl[], "MainLoadCellOffset[6]"=w460:sgl[], "MainLoadCellSensitivity[6]"=w459:sgl[], "BackupLoadCellCoefficient[6]"=w458:sgl[], "BackupLoadCellOffset[6]"=w457:sgl[], "BackupLoadCellSensitivity[6]"=w456:sgl[])  [unwired: 1 in, 5 out]
        n121 = Bundle By Name(cluster=w479, "Timestamp"=w477, "ReferenceId[6]"=w476, "ReferencePosition[6]"=w475, "ModbusSubnet[6]"=w474, "ModbusAddress[6]"=w473, "XPosition[6]"=w472, "YPosition[6]"=w471, "ZPosition[6]"=w470, "ILCUniqueId[6]"=w469, "ILCApplicationType[6]"=w468, "NetworkNodeType[6]"=w467, "ILCSelectedOptions[6]"=w466, "NetworkNodeOptions[6]"=w465, "MajorRevision[6]"=w464, "MinorRevision[6]"=w463, "ADCScanRate[6]"=w462, "MainLoadCellCoefficient[6]"=w461, "MainLoadCellOffset[6]"=w460, "MainLoadCellSensitivity[6]"=w459, "BackupLoadCellCoefficient[6]"=w458, "BackupLoadCellOffset[6]"=w457, "BackupLoadCellSensitivity[6]"=w456) -> (w478:T2)
        n122 = local write "ActuatorInfoEvent"(w478) -> ()
      }
      event User Event {
        n123 = event-data() -> ("Timestamp"=w492:dbl, "ReferenceId[6]"=w491:i16[], "ModbusSubnet[6]"=w490:i16[], "ModbusAddress[6]"=w489:i16[], "ILCUniqueId[6]"=w488:i64[], "ILCApplicationType[6]"=w487:i16[], "NetworkNodeType[6]"=w486:i16[], "MajorRevision[6]"=w485:i16[], "MinorRevision[6]"=w484:i16[], "MezzanineUniqueId[6]"=w483:i64[], "MezzanineFirmwareType[6]"=w482:i16[], "MezzanineMajorRevision[6]"=w481:i16[], "MezzanineMinorRevision[6]"=w480:i16[])  [unwired: 1 in, 5 out]
        n124 = Bundle By Name(cluster=w494, "Timestamp"=w492, "ReferenceId[6]"=w491, "ModbusSubnet[6]"=w490, "ModbusAddress[6]"=w489, "ILCUniqueId[6]"=w488, "ILCApplicationType[6]"=w487, "NetworkNodeType[6]"=w486, "MajorRevision[6]"=w485, "MinorRevision[6]"=w484, "MezzanineUniqueId[6]"=w483, "MezzanineFirmwareType[6]"=w482, "MezzanineMajorRevision[6]"=w481, "MezzanineMinorRevision[6]"=w480) -> (w493:T1)
        n125 = local write "MonitorInfoEvent"(w493) -> ()
      }
    }
    n126 = control-ref of="ActuatorInfoEvent"() -> (w321:refnum<vi>)
    n127 = control-ref of="MonitorInfoEvent"() -> (w312:refnum<vi>)
    n128 = property class="Clust (strict)"(reference=w312) -> (reference out=w296:refnum<vi>, error out=w309:errorcluster, "Controls[]"=w313:refnum<vi>[])  [unwired: 1 in]
    n129 = property class="Clust (strict)"(reference=w321) -> (reference out=w294:refnum<vi>, error out=w315:errorcluster, "Controls[]"=w316:refnum<vi>[])  [unwired: 1 in]
    n130 = Concatenate Strings("Events Data Type", "[6]" ("string")) -> (w305:string)
    n131 = call "Obtain Timestamp.vi"("error in (no error)"=w309, "ControlRefnumArray"=w313) -> ("error out"=w292:errorcluster, "Time Stamp"=→"Monitor Info Event Time Stamp":timestamp, "Array"=w301:refnum<vi>[])  [unwired: 7 in]
    n132 = call "Obtain Timestamp.vi"("error in (no error)"=w315, "ControlRefnumArray"=w316) -> ("error out"=w293:errorcluster, "Time Stamp"=→"Actuator Info Event Time Stamp":timestamp, "Array"=w310:refnum<vi>[])  [unwired: 7 in]
    n133 = String Subset(string=w305, offset (0)=0, length (rest)=8 ("length (rest)")) -> (substring=w304:string)
    n134 = Merge Errors(w293, w292) -> (w291:errorcluster)
    n135 = case shown="\"Monitor-\"" w304 {
      tunnel: w310 -> [_ w396]
      tunnel: [w328 w395] -> w306
      tunnel: w305 -> [w332 w394]
      tunnel: w301 -> [w329 _]
      tunnel: w291 -> [w326 w393]
      tunnel: [w327 w392] -> w290
      frame "Monitor-" {
        n136 = String Subset(string=w332, offset (0)=8) -> (substring=w330:string)  [unwired: 1 in]
        n137 = for {
          tunnel: w330 -> [w341]
          tunnel: w329 -> [w346] mode=indexing
          tunnel: [w334] -> w327
          tunnel: [w339] -> w328
          tunnel: w326 -> [w337]
          stop <- w343 stop-if-true
          n138 = property class="Ctl"(reference=w346, error in=w337) -> (reference out=w344:refnum<vi>, error out=w345:errorcluster, "Label.Text"=w340:string)
          n139 = Equal?(x=w341, y=w340) -> (x = y?=w343:bool)
          n140 = property class="Ctl"(reference=w344, error in=w345) -> (reference out=w338:refnum<vi>, error out=w342:errorcluster, "Value"=w347:variant)
          n141 = case shown="True" w343 {
            tunnel: w347 -> [_ w352]
            tunnel: w340 -> [_ _]
            tunnel: w342 -> [w350 w354]
            tunnel: [w350 w358] -> w335
            tunnel: [string[] [] w357] -> w339
            tunnel: w338 -> [w348 w356]
            tunnel: [w348 w355] -> w333
            frame False {
            }
            frame True {
              n142 = call <vilib>:"Get Type Information.vi"("error in (no error)"=w354, "Variant"=w352) -> ("error out"=w353:errorcluster, "Type"=w351:T7)  [unwired: 5 in, 3 out]
              n143 = case shown="Default" w351 {
                tunnel: w352 -> [w364 w374 w384]
                tunnel: [w360 w370 w379] -> w357
                tunnel: w353 -> [w363 w373 w382]
                tunnel: [w362 w372 w381] -> w358
                tunnel: w356 -> [w359 w369 w378]
                tunnel: [w359 w369 w378] -> w355
                frame "I32" {
                  n144 = Variant To Data(error in=w363, type=i32[] [], Variant=w364) -> (data=w361:i32[], error out=w362:errorcluster)
                  n145 = for {
                    tunnel: w361 -> [w366] mode=indexing
                    tunnel: [w367] -> w360 mode=indexing
                    n146 = Format Into String(format string="%d", w366) -> (resulting string=w367:string)  [unwired: 2 in, 1 out]
                  }
                }
                frame "Boolean" {
                  n147 = Variant To Data(error in=w373, type=bool[] [], Variant=w374) -> (data=w371:bool[], error out=w372:errorcluster)
                  n148 = for {
                    tunnel: w371 -> [w377] mode=indexing
                    tunnel: [w376] -> w370 mode=indexing
                    n149 = call "Boolean to String.vi"("BooleanValue"=w377) -> ("StringForm"=w376:string)  [unwired: 1 out]
                  }
                }
                frame Default {
                  n150 = Variant To Data(error in=w382, type=dbl[] [], Variant=w384) -> (data=w380:dbl[], error out=w381:errorcluster)
                  n151 = for {
                    tunnel: w380 -> [w386] mode=indexing
                    tunnel: [w385] -> w379 mode=indexing
                    n152 = Format Into String(format string="%f", w386) -> (resulting string=w385:string)  [unwired: 2 in, 1 out]
                  }
                }
              }
            }
          }
          n153 = Not A Number/Path/Refnum?(number/path/refnum=w333) -> (NaN/Path/Refnum?=w336:bool)
          n154 = case shown="False" w336 {
            tunnel: w335 -> [w390 w391]
            tunnel: [w389 w391] -> w334
            tunnel: w333 -> [w388 _]
            frame False {
              n155 = Close Reference(reference=w388, error in (no error)=w390) -> (error out=w389:errorcluster)
            }
            frame True {
            }
          }
        }
      }
      frame "", Default {
        n156 = for {
          tunnel: w394 -> [w404]
          tunnel: w396 -> [w409] mode=indexing
          tunnel: [w398] -> w392
          tunnel: [w402] -> w395
          tunnel: w393 -> [w397]
          stop <- w406 stop-if-true
          n157 = property class="Ctl"(reference=w409, error in=w397) -> (reference out=w407:refnum<vi>, error out=w408:errorcluster, "Label.Text"=w403:string)
          n158 = Equal?(x=w404, y=w403) -> (x = y?=w406:bool)
          n159 = property class="Ctl"(reference=w407, error in=w408) -> (reference out=w401:refnum<vi>, error out=w405:errorcluster, "Value"=w410:variant)
          n160 = case shown="True" w406 {
            tunnel: w410 -> [_ w420]
            tunnel: w403 -> [_ w419]
            tunnel: w405 -> [w413 w418]
            tunnel: [w413 w417] -> w399
            tunnel: [string[] [] w416] -> w402
            tunnel: w401 -> [w411 w415]
            tunnel: [w411 w414] -> w400
            frame False {
            }
            frame True {
              n161 = case shown="\" \"" w419 {
                tunnel: w420 -> [w426 w436 w446]
                tunnel: [w422 w432 w441] -> w416
                tunnel: w418 -> [w425 w435 w444]
                tunnel: [w424 w434 w443] -> w417
                tunnel: w415 -> [w421 w431 w440]
                tunnel: [w421 w431 w440] -> w414
                frame "ADCScanRate[6]", "ILCApplicationType[6]", "ILCSelectedOptions[6]", "ILCUniqueId[6]", "MajorRevision[6]", "MinorRevision[6]", "ModbusAddress[6]", "ModbusSubnet[6]" {
                  n162 = Variant To Data(error in=w425, type=i32[] [], Variant=w426) -> (data=w423:i32[], error out=w424:errorcluster)
                  n163 = for {
                    tunnel: w423 -> [w429] mode=indexing
                    tunnel: [w428] -> w422 mode=indexing
                    n164 = Format Into String(format string="%d", w429) -> (resulting string=w428:string)  [unwired: 2 in, 1 out]
                  }
                }
                frame " " {
                  n165 = Variant To Data(error in=w435, type=bool[] [], Variant=w436) -> (data=w433:bool[], error out=w434:errorcluster)
                  n166 = for {
                    tunnel: w433 -> [w439] mode=indexing
                    tunnel: [w438] -> w432 mode=indexing
                    n167 = call "Boolean to String.vi"("BooleanValue"=w439) -> ("StringForm"=w438:string)  [unwired: 1 out]
                  }
                }
                frame "", Default {
                  n168 = Variant To Data(error in=w444, type=dbl[] [], Variant=w446) -> (data=w442:dbl[], error out=w443:errorcluster)
                  n169 = for {
                    tunnel: w442 -> [w449] mode=indexing
                    tunnel: [w448] -> w441 mode=indexing
                    n170 = Format Into String(format string="%f", w449) -> (resulting string=w448:string)  [unwired: 2 in, 1 out]
                  }
                }
              }
            }
          }
          n171 = Close Reference(reference=w400, error in (no error)=w399) -> (error out=w398:errorcluster)
        }
      }
    }
    n172 = call "PlaceDataInControls.vi"("error in (no error)"=w290, "Variant"=w307, "DataArray"=w306, "ControlNamesArray"=string[] ["E1", "E2", "E3", "E4", "E5", "E6"]) -> ("error out"=w297:errorcluster)  [unwired: 7 in]
    n173 = Not A Number/Path/Refnum?(number/path/refnum=w296) -> (NaN/Path/Refnum?=w298:bool)
    n174 = case shown="False" w298 {
      tunnel: w297 -> [w502 w503]
      tunnel: [w501 w503] -> w300
      tunnel: w296 -> [w500 _]
      frame False {
        n175 = Close Reference(reference=w500, error in (no error)=w502) -> (error out=w501:errorcluster)
      }
      frame True {
      }
    }
    n176 = Not A Number/Path/Refnum?(number/path/refnum=w294) -> (NaN/Path/Refnum?=w299:bool)
    n177 = case shown="False" w299 {
      tunnel: w300 -> [w498 w499]
      tunnel: [w497 w499] -> w295
      tunnel: w294 -> [w496 _]
      frame False {
        n178 = Close Reference(reference=w496, error in (no error)=w498) -> (error out=w497:errorcluster)
      }
      frame True {
      }
    }
  }
  n179 = while {
    tunnel: w78 -> [w511]
    tunnel: [w509] -> _
    shift-right: [w507] -> _
    shift-left: i32[] [0, 0, 0, 0, 0, 0] -> [w508]
    shift-right: [w505] -> _
    shift-left: T5."DetailedState_DetailedStates_OfflineState" ("y") -> [w506]
    tunnel: [errorcluster {"status"=FALSE, "code"=0, "source"=""} ("error constant")] -> w13
    stop <- w510 stop-if-true
    n180 = event shown="[0] <Detailed State Event>: User Event" {
      selector: w511 -> [_ _ _ _ _ _ _ _ _]
      dyn-events: [_ _ _ _ _ _ _ _ _] -> w509
      timeout: _ -> [_ _ _ _ _ _ _ _ _]
      tunnel: [w515 _ _ _ _ _ _ _ _] -> w510
      tunnel: w508 -> [w514 w519 w535 w552 w582 w590 w616 w648 w674]
      tunnel: [w514 w519 w535 w552 w582 w590 w616 w648 w674] -> w507
      tunnel: w506 -> [_ w520 w536 w554 w581 w592 w618 w653 w679]
      tunnel: [w512 w520 w536 w554 w581 w592 w618 w653 w679] -> w505
      event User Event {
        n181 = event-data() -> ("DetailedState"=w512:T5)  [unwired: 1 in, 6 out]
        n182 = Equal?(x=w512, y=T5."DetailedState_DetailedStates_OfflineState") -> (x = y?=w515:bool)
      }
      event "EnableHardpointCorrectionButton": Value Change {
        n183 = event-data() -> ()  [unwired: 1 in, 1 out]
        n184 = control-ref of="EnableHardpointCorrectionButton"() -> (w521:refnum<vi>)
        n185 = control-ref of="DisableHardpointCorrectionButton"() -> (w517:refnum<vi>)
        n186 = Equal?(x=T5."DetailedState_DetailedStates_ActiveEngineeringState", y=w520) -> (x = y?=w523:bool)
        n187 = And(x="EnableHardpointCorrectionButton", y=w523) -> (x .and. y?=w518:bool)
        n188 = case shown="True" w518 {
          tunnel: w521 -> [_ w532]
          tunnel: w517 -> [_ w531]
          frame False {
            # "State error that action is unavailable as system is not in \nActive Engineering State"
          }
          frame True {
            n189 = call "m1m3_issueCommand_EnableHardpointCorrections.vi"("command_EnableHardpointCorrections_Ctl"=T8 {"EnableHardpointCorrections"=TRUE}) -> ("error out"=w528:errorcluster, "function return"=w525:i32)  [unwired: 8 in, 1 out]
            n190 = property class="Bool"(reference=w532, "Visible"=FALSE) -> ()  [unwired: 1 in, 2 out]
            n191 = property class="Bool"(reference=w531, "Visible"=TRUE) -> ()  [unwired: 1 in, 2 out]
            n192 = Bundle By Name(cluster=cluster{"cmdSeqNum":i32, "timeout":u32} {"cmdSeqNum"=0, "timeout"=100} ("waitComplete_Ctl"), "cmdSeqNum"=w525) -> (w524:cluster{"cmdSeqNum":i32, "timeout":u32})
            n193 = call "m1m3_waitForCompletion_EnableHardpointCorrections.vi"("error in (no error)"=w528, "waitComplete_Ctl"=w524) -> ("error out"=w527:errorcluster)  [unwired: 7 in, 2 out]
            n194 = call <vilib>:"Simple Error Handler.vi"("error in (no error)"=w527) -> ()  [unwired: 4 in, 5 out]
          }
        }
      }
      event "DisableHardpointCorrectionButton": Value Change {
        n195 = event-data() -> ()  [unwired: 1 in, 1 out]
        n196 = control-ref of="EnableHardpointCorrectionButton"() -> (w537:refnum<vi>)
        n197 = control-ref of="DisableHardpointCorrectionButton"() -> (w538:refnum<vi>)
        n198 = Equal?(x=T5."DetailedState_DetailedStates_ActiveEngineeringState", y=w536) -> (x = y?=w541:bool)
        n199 = And(x="DisableHardpointCorrectionButton", y=w541) -> (x .and. y?=w539:bool)
        n200 = case shown="True" w539 {
          tunnel: w538 -> [_ w547]
          tunnel: w537 -> [_ w545]
          frame False {
          }
          frame True {
            n201 = call "m1m3_issueCommand_DisableHardpointCorrections.vi"("command_DisableHardpointCorrections_Ctl"=T9 {"DisableHardpointCorrections"=TRUE}) -> ("error out"=w550:errorcluster, "function return"=w543:i32)  [unwired: 8 in, 1 out]
            n202 = property class="Bool"(reference=w545, "Visible"=TRUE) -> ()  [unwired: 1 in, 2 out]
            n203 = property class="Bool"(reference=w547, "Visible"=FALSE) -> ()  [unwired: 1 in, 2 out]
            n204 = Bundle By Name(cluster=cluster{"cmdSeqNum":i32, "timeout":u32} {"cmdSeqNum"=0, "timeout"=100} ("waitComplete_Ctl"), "cmdSeqNum"=w543) -> (w542:cluster{"cmdSeqNum":i32, "timeout":u32})
            n205 = call "m1m3_waitForCompletion_DisableHardpointCorrections.vi"("error in (no error)"=w550, "waitComplete_Ctl"=w542) -> ("error out"=w549:errorcluster)  [unwired: 7 in, 2 out]
            n206 = call <vilib>:"Simple Error Handler.vi"("error in (no error)"=w549) -> ()  [unwired: 4 in, 5 out]
          }
        }
      }
      event "HardpointMotionButton": Value Change {
        n207 = event-data() -> ()  [unwired: 1 in, 1 out]
        n208 = case shown="True" "HardpointMotionButton" {
          frame False {
          }
          frame True {
            # "command_MoveHardpointActuators_Ctl"
            n209 = Insert Into Array(array=i32[] [], index=0, new element="Input 1") -> (w574:i32[])
            n210 = Insert Into Array(array=w574, index=1, new element="Input 2") -> (w572:i32[])
            n211 = Insert Into Array(array=w572, index=2, new element="Input 3") -> (w570:i32[])
            n212 = Insert Into Array(array=w570, index=3, new element="Input 4") -> (w568:i32[])
            n213 = Insert Into Array(array=w568, index=4, new element="Input 5") -> (w566:i32[])
            n214 = Insert Into Array(array=w566, index=5, new element="Input 6") -> (w560:i32[])
            n215 = Bundle By Name(cluster=T10 {"Steps[6]"=[0, 0, 0, 0, 0, 0]} ("command_MoveHardpointActuators_Ctl"), "Steps[6]"=w560) -> (w579:T10)
            n216 = call "m1m3_issueCommand_MoveHardpointActuators.vi"("command_MoveHardpointActuators_Ctl"=w579) -> ("error out"=w558:errorcluster, "function return"=w556:i32)  [unwired: 8 in, 1 out]
            n217 = Bundle By Name(cluster=cluster{"cmdSeqNum":i32, "timeout":u32} {"cmdSeqNum"=0, "timeout"=100} ("waitComplete_Ctl"), "cmdSeqNum"=w556) -> (w555:cluster{"cmdSeqNum":i32, "timeout":u32})
            n218 = call "m1m3_waitForCompletion_MoveHardpointActuators.vi"("error in (no error)"=w558, "waitComplete_Ctl"=w555) -> ("error out"=w559:errorcluster)  [unwired: 7 in, 2 out]
            n219 = call <vilib>:"Simple Error Handler.vi"("error in (no error)"=w559) -> ()  [unwired: 4 in, 5 out]
          }
        }
      }
      event "StopHardpointMotion": Value Change {
        n220 = event-data() -> ()  [unwired: 1 in, 6 out]
        n221 = case shown="True" "StopHardpointMotion" {
          frame False {
          }
          frame True {
            n222 = call "m1m3_issueCommand_StopHardpointMotion.vi"("command_StopHardpointMotion_Ctl"=T11 {"StopHardpointMotion"=TRUE}) -> ("error out"=w584:errorcluster, "function return"=w586:i32)  [unwired: 8 in, 1 out]
            n223 = Bundle By Name(cluster=cluster{"cmdSeqNum":i32, "timeout":u32} {"cmdSeqNum"=0, "timeout"=100} ("waitComplete_Ctl"), "cmdSeqNum"=w586) -> (w585:cluster{"cmdSeqNum":i32, "timeout":u32})
            n224 = call "m1m3_waitForCompletion_StopHardpointMotion.vi"("error in (no error)"=w584, "waitComplete_Ctl"=w585) -> ("error out"=w588:errorcluster)  [unwired: 7 in, 2 out]
            n225 = call <vilib>:"Simple Error Handler.vi"("error in (no error)"=w588) -> ()  [unwired: 4 in, 5 out]
          }
        }
      }
      event "EnableHardpointChaseButton": Value Change {
        n226 = event-data() -> ()  [unwired: 1 in, 6 out]
        n227 = local read "EnableActuatorId"() -> (w591:string)
        n228 = case shown="True" "EnableHardpointChaseButton" {
          tunnel: w591 -> [_ w594]
          frame False {
          }
          frame True {
            n229 = case shown="\"1\", Default" w594 {
              selector: w594 -> [w606 _]
              tunnel: i32[] [] -> [w608 w610]
              tunnel: [w607 w609] -> w595
              frame "1", Default {
                n230 = Decimal String To Number(string=w606) -> (number=w605:i32)  [unwired: 2 in, 1 out]
                n231 = Insert Into Array(array=w608, new element=w605) -> (w607:i32[])  [unwired: 1 in]
              }
              frame "ALL" {
                n232 = for {
                  N: 6 -> [_]
                  shift-right: [w614] -> w609
                  shift-left: w610 -> [w615]
                  i -> [w612]
                  n233 = Increment(x=w612) -> (x+1=w613:i32)
                  n234 = Insert Into Array(array=w615, index=w612, new element=w613) -> (w614:i32[])
                }
              }
            }
            n235 = for {
              tunnel: w595 -> [w604] mode=indexing
              n236 = Bundle By Name(cluster=T12 {"HardpointActuator"=0} ("command_EnableHardpointChase_Ctl"), "HardpointActuator"=w604) -> (w602:T12)
              n237 = call "m1m3_issueCommand_EnableHardpointChase.vi"("command_EnableHardpointChase_Ctl"=w602) -> ("error out"=w597:errorcluster, "function return"=w599:i32)  [unwired: 8 in, 1 out]
              n238 = Bundle By Name(cluster=cluster{"cmdSeqNum":i32, "timeout":u32} {"cmdSeqNum"=0, "timeout"=100} ("waitComplete_Ctl"), "cmdSeqNum"=w599) -> (w598:cluster{"cmdSeqNum":i32, "timeout":u32})
              n239 = call "m1m3_waitForCompletion_EnableHardpointChase.vi"("error in (no error)"=w597, "waitComplete_Ctl"=w598) -> ("error out"=w601:errorcluster)  [unwired: 7 in, 2 out]
              n240 = call <vilib>:"Simple Error Handler.vi"("error in (no error)"=w601) -> ()  [unwired: 4 in, 5 out]
            }
          }
        }
      }
      event "DisableHardpointChaseButton": Value Change {
        n241 = event-data() -> ()  [unwired: 1 in, 6 out]
        n242 = local read "EnableActuatorId"() -> (w617:string)
        n243 = case shown="True" "DisableHardpointChaseButton" {
          tunnel: w617 -> [_ w620]
          frame False {
          }
          frame True {
            n244 = case shown="\"1\", Default" w620 {
              selector: w620 -> [w624 _]
              tunnel: i32[] [] -> [w626 w628]
              tunnel: [w625 w627] -> w621
              frame "1", Default {
                n245 = Decimal String To Number(string=w624) -> (number=w623:i32)  [unwired: 2 in, 1 out]
                n246 = Insert Into Array(array=w626, new element=w623) -> (w625:i32[])  [unwired: 1 in]
              }
              frame "ALL" {
                n247 = for {
                  N: 6 -> [_]
                  shift-right: [w632] -> w627
                  shift-left: w628 -> [w633]
                  i -> [w630]
                  n248 = Increment(x=w630) -> (x+1=w631:i32)
                  n249 = Insert Into Array(array=w633, index=w630, new element=w631) -> (w632:i32[])
                }
              }
            }
            n250 = for {
              tunnel: w621 -> [w639] mode=indexing
              n251 = Bundle By Name(cluster=T13 {"HardpointActuator"=0} ("command_DisableHardpointChase_Ctl"), "HardpointActuator"=w639) -> (w640:T13)
              n252 = call "m1m3_issueCommand_DisableHardpointChase.vi"("command_DisableHardpointChase_Ctl"=w640) -> ("error out"=w634:errorcluster, "function return"=w636:i32)  [unwired: 8 in, 1 out]
              n253 = Bundle By Name(cluster=cluster{"cmdSeqNum":i32, "timeout":u32} {"cmdSeqNum"=0, "timeout"=100} ("waitComplete_Ctl"), "cmdSeqNum"=w636) -> (w635:cluster{"cmdSeqNum":i32, "timeout":u32})
              n254 = call "m1m3_waitForCompletion_DisableHardpointChase.vi"("error in (no error)"=w634, "waitComplete_Ctl"=w635) -> ("error out"=w638:errorcluster)  [unwired: 7 in, 2 out]
              n255 = call <vilib>:"Simple Error Handler.vi"("error in (no error)"=w638) -> ()  [unwired: 4 in, 5 out]
            }
          }
        }
      }
      event "PositionHardpointsButton": Value Change {
        n256 = event-data() -> ()  [unwired: 1 in, 1 out]
        n257 = for {
          tunnel: w648 -> [w658] mode=indexing
          shift-right: [w654] -> w650
          shift-left: TRUE -> [w655]
          n258 = Equal?(x=0, y=w658) -> (x = y?=w656:bool)
          n259 = And(x=w655, y=w656) -> (x .and. y?=w654:bool)
        }
        n260 = local read "X Position Input"() -> (w647:dbl)
        n261 = local read "Y Position Input"() -> (w646:dbl)
        n262 = local read "Z Position Input"() -> (w645:dbl)
        n263 = local read "X Rotation Input"() -> (w644:dbl)
        n264 = local read "Y Rotation Input"() -> (w643:dbl)
        n265 = local read "Z Rotation Input"() -> (w642:dbl)
        n266 = And(x="PositionHardpointsButton", y=w650) -> (x .and. y?=w651:bool)
        n267 = case shown="True" w651 {
          tunnel: w644 -> [_ w664]
          tunnel: w643 -> [_ w662]
          tunnel: w642 -> [_ w663]
          tunnel: w647 -> [_ w666]
          tunnel: w646 -> [_ w659]
          tunnel: w645 -> [_ w665]
          frame False {
            # "Send error message that not all \nHP are still"
          }
          frame True {
            n268 = Bundle By Name(cluster=T14 {"XPosition"=0.0, "YPosition"=0.0, "ZPosition"=0.0, "XRotation"=0.0, "YRotation"=0.0, "ZRotation"=0.0} ("command_PositionM1M3_Ctl"), "XPosition"=w666, "YPosition"=w659, "ZPosition"=w665, "XRotation"=w664, "YRotation"=w662, "ZRotation"=w663) -> (w660:T14)
            n269 = call "m1m3_issueCommand_PositionM1M3.vi"("command_PositionM1M3_Ctl"=w660) -> ("error out"=w661:errorcluster)  [unwired: 8 in, 2 out]
            n270 = call <vilib>:"Simple Error Handler.vi"("error in (no error)"=w661) -> ()  [unwired: 4 in, 5 out]
          }
        }
      }
      event "TranslateHardpointsButton": Value Change {
        n271 = event-data() -> ()  [unwired: 1 in, 1 out]
        n272 = for {
          tunnel: w674 -> [w684] mode=indexing
          shift-right: [w680] -> w677
          shift-left: TRUE -> [w681]
          n273 = Equal?(x=0, y=w684) -> (x = y?=w682:bool)
          n274 = And(x=w681, y=w682) -> (x .and. y?=w680:bool)
        }
        n275 = local read "Y Position Input"() -> (w672:dbl)
        n276 = local read "X Rotation Input"() -> (w670:dbl)
        n277 = local read "Y Rotation Input"() -> (w669:dbl)
        n278 = local read "X Position Input"() -> (w673:dbl)
        n279 = local read "Z Position Input"() -> (w671:dbl)
        n280 = local read "Z Rotation Input"() -> (w668:dbl)
        n281 = And(x="TranslateHardpointsButton", y=w677) -> (x .and. y?=w675:bool)
        n282 = case shown="True" w675 {
          tunnel: w673 -> [_ w691]
          tunnel: w672 -> [_ w690]
          tunnel: w671 -> [_ w689]
          tunnel: w670 -> [_ w688]
          tunnel: w668 -> [_ w687]
          tunnel: w669 -> [_ w686]
          frame False {
            # "Send error message that not all HP\nare still, so not possible"
          }
          frame True {
            n283 = Bundle By Name(cluster=T15 {"XTranslation"=0.0, "YTranslation"=0.0, "ZTranslation"=0.0, "XRotation"=0.0, "YRotation"=0.0, "ZRotation"=0.0} ("command_TranslateM1M3_Ctl"), "XTranslation"=w691, "YTranslation"=w690, "ZTranslation"=w689, "XRotation"=w688, "YRotation"=w686, "ZRotation"=w687) -> (w685:T15)
            n284 = call "m1m3_issueCommand_TranslateM1M3.vi"("command_TranslateM1M3_Ctl"=w685) -> ("error out"=w693:errorcluster)  [unwired: 8 in, 2 out]
            n285 = call <vilib>:"Simple Error Handler.vi"("error in (no error)"=w693) -> ()  [unwired: 4 in, 5 out]
          }
        }
      }
    }
  }
  n286 = control-ref of="This VI"() -> (w24:refnum<vi>)
  n287 = control-ref of="This VI"() -> (w23:refnum<vi>)
  n288 = call "Close References.vi"("error in (no error)"=w19, "VI Refnum"=w24, "Variant"=w25) -> ("error out"=w67:errorcluster)  [unwired: 8 in]
  n289 = call "Close References.vi"("error in (no error)"=w22, "VI Refnum"=w23, "Variant"=w21) -> ("error out"=w14:errorcluster)  [unwired: 8 in]
  n290 = Not A Number/Path/Refnum?(number/path/refnum=w17) -> (NaN/Path/Refnum?=w18:bool)
  n291 = Merge Errors(w67, w14, w13) -> (w16:errorcluster)
  n292 = case shown="False" w18 {
    tunnel: w17 -> [w696 _]
    tunnel: w16 -> [w695 w697]
    tunnel: [w694 w697] -> w15
    frame False {
      n293 = Unregister For Events(event registration refnum=w696, error in=w695) -> (error out=w694:errorcluster)
    }
    frame True {
    }
  }
  n294 = call <vilib>:"Simple Error Handler.vi"("error in (no error)"=w15) -> ()  [unwired: 4 in, 5 out]
